vi "DQMH Load API Tester.vi"(7 "Application reference":refnum<vi>, 8 "error in (no error)":errorcluster, 11 "Module Disk Path":path) -> (0 "error out":errorcluster)   [LabVIEW 2022 SP3, in "hse-dqmh-dynamicrequesters.lvlib"]
doc: "Calls the \"Load Module\" request VI of the module in <b>path</b>\n\n____\nHAMPEL SOFTWARE ENGINEERING v3.8.0 (2023-12-18 14:41)"
uses:
  hse-dqmh-dynamicrequesters.lvlib
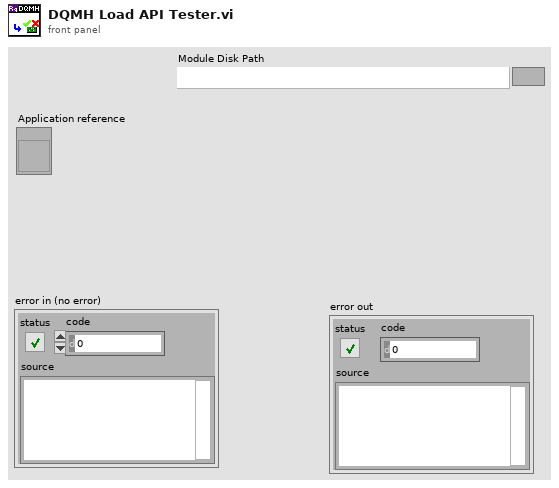
[diagram p1: front panel]
types:
  T1 = enum32{"Bad", "Idle", "Run top level", "Running"}
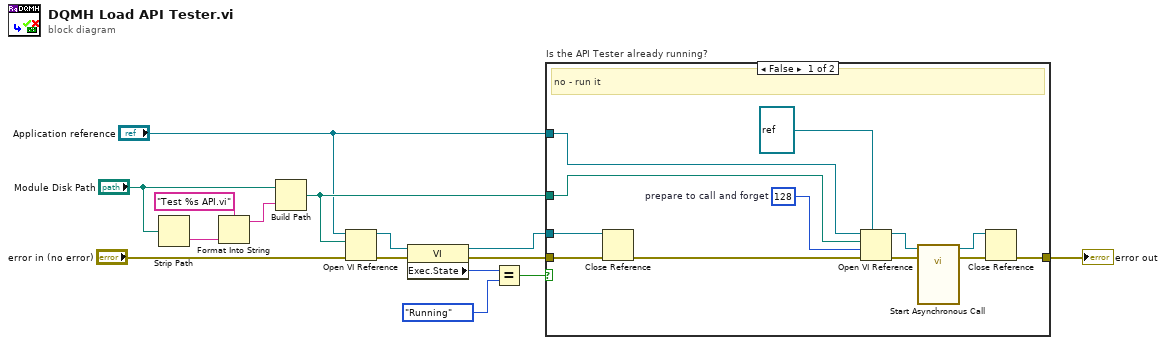
[diagram p0: block diagram]
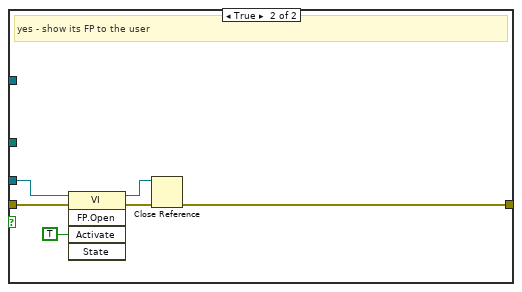
[diagram p2: hidden frame]
diagram:
  n1 = Strip Path(path="Module Disk Path") -> (name=w11:string)  [unwired: 1 out]
  n2 = Format Into String(format string="Test %s API.vi" ("name or relative path"), w11) -> (resulting string=w13:string)  [unwired: 2 in, 1 out]
  n3 = Build Path(base path="Module Disk Path", name or relative path=w13) -> (appended path=w9:path)
  n4 = Open VI Reference(application reference (local)="Application reference", vi path=w9, error in (no error)="error in (no error)") -> (vi reference=w7:refnum<vi>, error out=w1:errorcluster)  [unwired: 3 in]
  n5 = property class="VI"(reference=w7, error in=w1) -> (reference out=w3:refnum<vi>, error out=w2:errorcluster, "Exec.State"=w6:T1)
  n6 = Equal?(x=w6, y=T1."Running" ("Execution:State")) -> (x = y?=w4:bool)
  n7 = case "Is the API Tester already running?" shown="False" w4 {
    tunnel: w3 -> [w26 w33]
    tunnel: w2 -> [w27 w30]
    tunnel: [w17 w28] -> w10
    tunnel: w9 -> [w23 _]
    tunnel: "Application reference" -> [w22 _]
    frame False {
      w16 = 128  # prepare to call and forget
      # "no - run it"
      n8 = Close Reference(reference=w26, error in (no error)=w27) -> (error out=w24:errorcluster)
      n9 = Open VI Reference(type specifier VI Refnum (for type only)=refnum<vi> refnum, application reference (local)=w22, vi path=w23, options=w16, error in (no error)=w24) -> (vi reference=w20:refnum<vi>, error out=w21:errorcluster)  [unwired: 1 in]
      n10 = call-by-ref "Start Asynchronous Call"(reference=w20, error in=w21) -> (reference out=w19:refnum<vi>, error out=w18:errorcluster)  [unwired: 12 in]
      n11 = Close Reference(reference=w19, error in (no error)=w18) -> (error out=w17:errorcluster)
    }
    frame True {
      # "yes - show its FP to the user"
      n12 = invoke class="VI" method="FP.Open"(reference=w33, error in=w30, "Activate"=TRUE ("Activate?")) -> (reference out=w31:refnum<vi>, error out=w29:errorcluster)  [unwired: 2 in, 3 out]
      n13 = Close Reference(reference=w31, error in (no error)=w29) -> (error out=w28:errorcluster)
    }
  }
  "error out" <- w10
